vi "Get Terminal Names.vi"(7 "Input Terms[]":refnum<vi>[](array[refnum])) -> (6 "Type":T1[](array[typedef]), 10 "Name":string[](array[string]))   [LabVIEW 2018]
doc: "Created by VI-Tech"
uses:
  <vilib>/Utility/Data Type/Type Definitions/Data Type.ctl
  <vilib>/addons/analyzer/_analyzerutils.llb/VIAnUtil Check Type If ErrClust.vi
  <vilib>/Utility/Data Type/NI_Data Type.lvlib
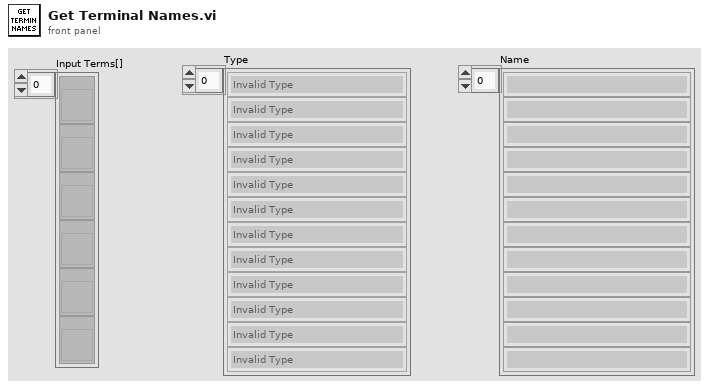
[diagram p1: front panel]
types:
  T1 = typedef "NI_Data Type.lvlib/Data Type.ctl" = enum8{"Invalid Type", "Void", "I8", "I16", "I32", "I64", "U8", "U16", "U32", "U64", "Single Float", "Double Float", "Extended Float", "Single Complex", "Double Complex", "Extended Complex", "Enum U8", "Enum U16", "Enum U32", "Enum U64", "Single Float With Unit", "Double Float With Unit", "Extended Float With Unit", "Single Complex with Unit", "Double Complex with Unit", "Extended Complex with Unit", "Boolean", "String", "Path", "Picture", "Tag", "Array", "Cluster", "Variant", "LV Variant", "Waveform", "Timestamp", "Digital Waveform", "Digital Data", "ExpressData", "Refnum", "External Data", "VI", "Poly VI", "LabVIEW Class Instance", "Fixed Point"}
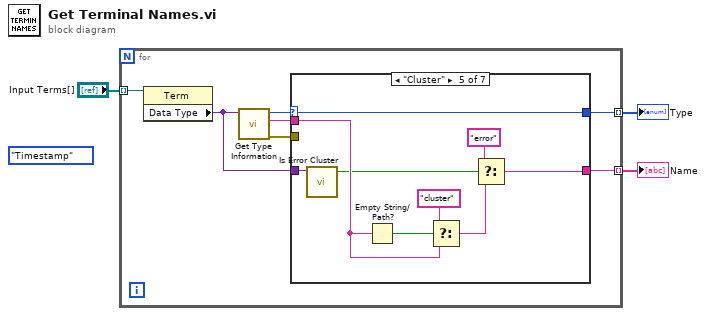
[diagram p0: block diagram]
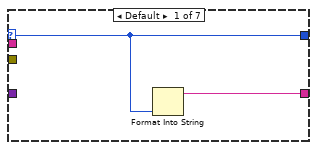
[diagram p2: hidden frame]
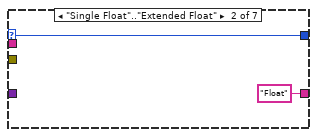
[diagram p3: hidden frame]
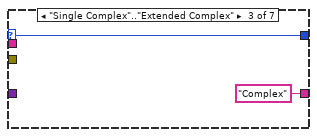
[diagram p4: hidden frame]
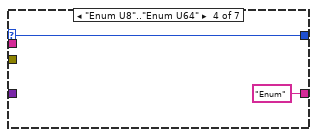
[diagram p5: hidden frame]
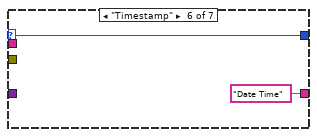
[diagram p6: hidden frame]
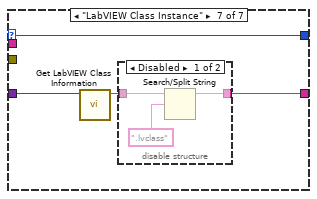
[diagram p7: hidden frame]
diagram:
  (unwired) Data_Type."Timestamp" ("Type")
  n1 = for {
    tunnel: "Input Terms[]" -> [w10] mode=indexing
    tunnel: [w6] -> w2 mode=indexing
    tunnel: [w8] -> w3 mode=indexing
    n2 = property class="Term"(reference=w10) -> ("Data Type"=w5:variant)  [unwired: 1 in, 2 out]
    n3 = call <vilib>:"Get Type Information.vi"("Variant"=w5) -> ("error out"=w7:errorcluster, "Name"=w4:string, "Type"=w9:T1)  [unwired: 6 in, 2 out]
    n4 = case shown="\"Cluster\"" w9 {
      selector: w9 -> [w12 w14 w16 w18 w27 w29 w32]
      tunnel: [w12 w14 w16 w18 w27 w29 w32] -> w8
      tunnel: w7 -> [_ _ _ _ _ _ _]
      tunnel: [w11 "Float" ("LabVIEW class file name") "Complex" ("LabVIEW class file name") "Enum" ("LabVIEW class file name") w26 "Date Time" ("LabVIEW class file name") w30] -> w6
      tunnel: w5 -> [_ _ _ _ w25 _ w33]
      tunnel: w4 -> [_ _ _ _ w22 _ _]
      frame Default {
        n5 = Format Into String(w12) -> (resulting string=w11:string)  [unwired: 3 in, 1 out]
      }
      frame "Single Float".."Extended Float" {
      }
      frame "Single Complex".."Extended Complex" {
      }
      frame "Enum U8".."Enum U64" {
      }
      frame "Cluster" {
        n6 = call "Is Error Cluster.vi"("variant"=w25) -> ("is error cluster?"=w19:bool)  [unwired: 9 in, 1 out]
        n7 = Empty String/Path?(string/path=w22) -> (empty?=w23:bool)
        n8 = Select(t="cluster", s=w23, f=w22) -> (s? t:f=w21:string)
        n9 = Select(t="error", s=w19, f=w21) -> (s? t:f=w26:string)
      }
      frame "Timestamp" {
      }
      frame "LabVIEW Class Instance" {
        n10 = call <vilib>:"Get LabVIEW Class Information.vi"("Variant"=w33) -> ("LabVIEW Class File Name"=w31:string)  [unwired: 8 in, 2 out]
        n11 = disable-structure shown="Disabled" {
          disable-tunnel: w31 -> [w35 w37]
          disable-tunnel: [w34 w37] -> w30
          frame Disabled {
            n12 = Search/Split String(string=w35, search string/char (-)=".lvclass") -> (substring before match=w34:string)  [unwired: 1 in, 2 out]
          }
          frame Enabled {
            # "Keep the .lvclass\nin the search. For\nclass results"
          }
        }
      }
    }
  }
  "Type" <- w3
  "Name" <- w2
